vi "ChangeFileExtension.vi"(9 "NewExtenion":string, 11 "In FileName":path) -> (3 "Out FileName":path)   [LabVIEW 2019]
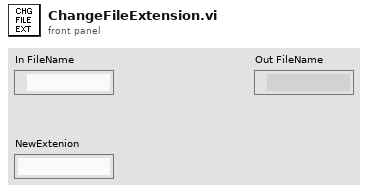
[diagram p1: front panel]
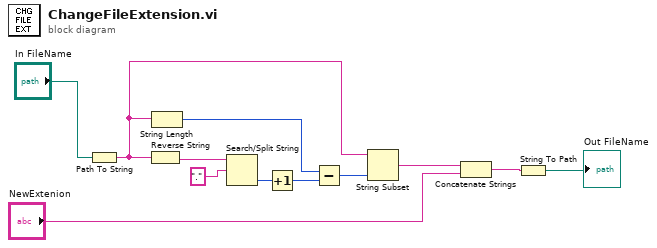
[diagram p0: block diagram]
diagram:
  n1 = Path To String(path="In FileName") -> (string=w8:string)
  n2 = Reverse String(1:w8) -> (0:w11:string)
  n3 = String Length(string=w8) -> (length=w9:i32)
  n4 = Search/Split String(string=w11, search string/char (-)=".") -> (offset of match=w7:i32)  [unwired: 1 in, 2 out]
  n5 = Increment(x=w7) -> (x+1=w6:i32)
  n6 = Subtract(x=w9, y=w6) -> (x-y=w5:i32)
  n7 = String Subset(string=w8, length (rest)=w5) -> (substring=w4:string)  [unwired: 1 in]
  n8 = Concatenate Strings(w4, "NewExtenion") -> (w2:string)
  n9 = String To Path(string=w2) -> (path=→"Out FileName":path)
